vi "SDG60CreateArbWaveformFlatten3.vi"(4 "WFM Source":u16(ring) items=["Single file", "Split files", "Array"], 5 "WFM (Column) Number":i32, 6 "Array WFM":i16[](array[numeric])=[1000, 2000, 3000, 4000, 5000, 6000, 7000, 8000], 7 "WFM Length":i32=15, 8 "error in (no error)":errorcluster, 9 "Timeout (40000 ms)":u32=40000, 10 "Waveform Name (\"wave1\")":string="wave1", 11 "VISA resource name":refnum<visa-resource-name>="USB0::0xF4EC::0x1101::SDG6XEBC5R0119::INSTR") -> (0 "error out":errorcluster, 3 "VISA resource name out":refnum<visa-resource-name>)   [LabVIEW 2018]
doc: "Creates and saves an arbitrary (user-defined) waveform in non-volatile memory, then selects it for output."
uses:
  <vilib>/Utility/file.llb/Read From Spreadsheet File (I64).vi
panel:
  out "Check String":string
  out "WFM to arr time":dbl
  out "Arr to str time":dbl
  out "Upload time":dbl
  out "Total time":dbl
  out "Attempts 0: First":i32
  in  "WFM Path":path=path "C:/Data/_SoftDevelopment/SDG6000/WFMTst20E6PtsInt.txt"
  # "Same vi as with suppliers example, but incorrect negative case removed.\nInstead calculating twos complement explicitly for negative values.\nThe input range for ARB data is: -32767..+32767 (must be integers)\n\nC1 hardcoded as needs to have a channel\nassigned to be uploaded. \nCan then be selected for either channel\n\nUpon overwrite of name with new WFM, still needs to be selected\notherwise will still use old WFM. If WFM has been selected, and then gets deleted off \nC drive, will still output WFM on that channel\n\nTesting uploads of large WFMS.\n8M: All ok, can have 2 separate WFMs on 2 channels and upload more\n16M: Can have 2 separate WFMs on 2 channels, storage space limits 3rd upload\n          of 16M points, but can upload 8M and switch fine between them all.\n20M: Can have 20M on both channels, but then no storage space to upload third\n\nVi will write the file with a small (16B bin file on device) file (overwriting any WFM \n           preciviously with that name),  then write the WFM selected with the one chosen to \n           upload.  This means you don't need to clear space off the device, as long as the \n           name of the WFM is already on the device. Provided it is that file that is the storage \n           issue. If a new name is chosen, then will have to manually delete the old WFM.\n\nIf too large a waveform is uploaded, generator will crash requiring manual power cycle\n\nIf storage full, will beep on machine-say storage full, but not give any error through \nlabview. Waveform won't ovewrite others when uploading\n\nSingle pixel test, (osciiloscope limited), for 20M points, the single pixel did go high, Pk-Pk on \nscope was 3.6V when should be 4.0 Vpp. This may be down to the scopes 200MHz resolution\nas the width of the of peak on the scope is ~350ns"
  # "Need to set name to be number. not string"
  # "Max  20E6 (decimal)"
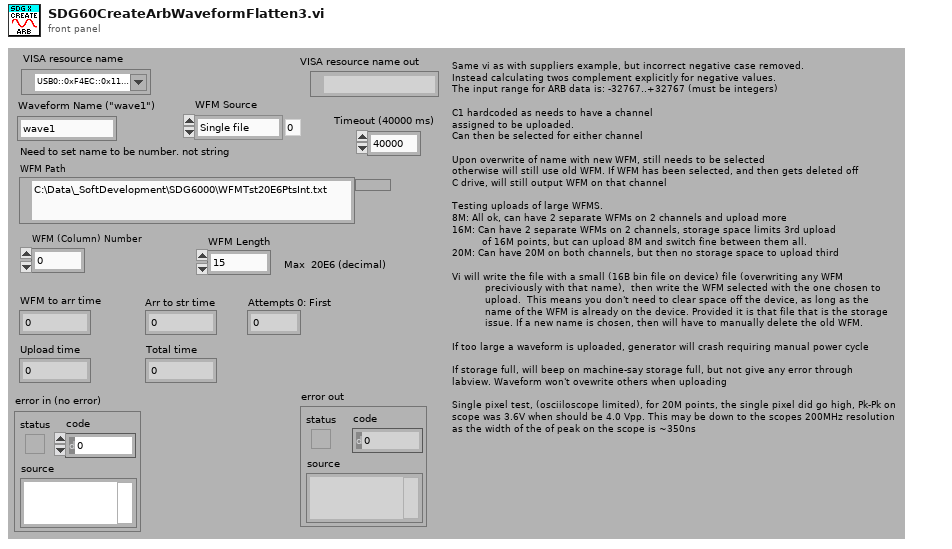
[diagram p1: front panel]
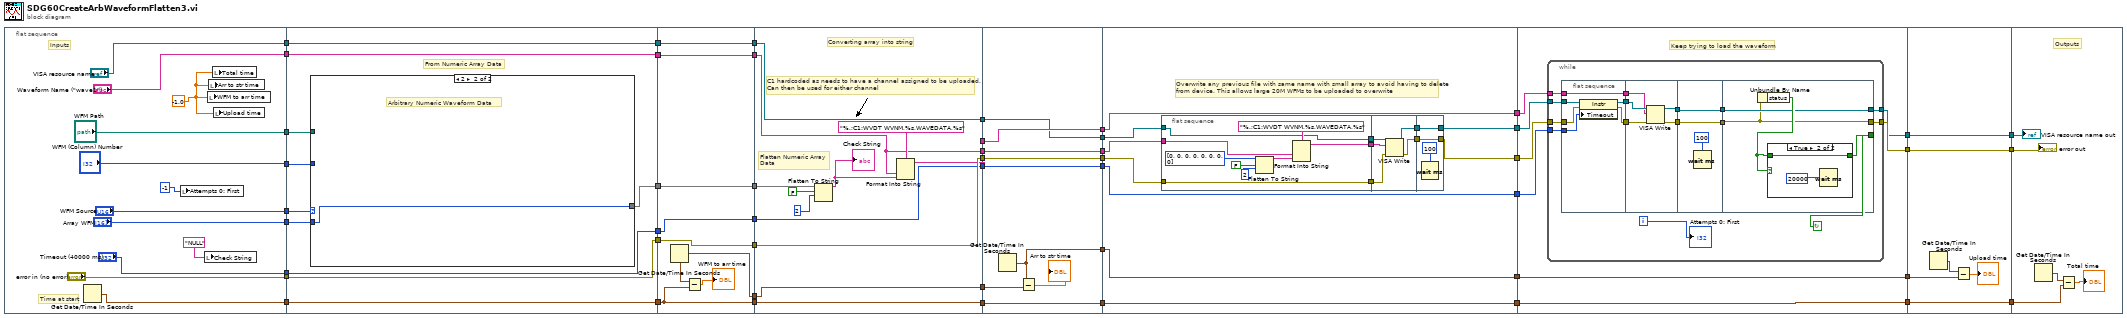
[diagram p0: block diagram]
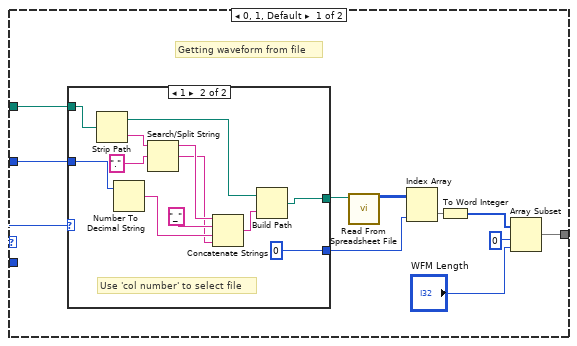
[diagram p2: hidden frame]
diagram:
  n1 = flat-sequence {
    tunnel: ["WFM Source"] -> w49
    tunnel: ["Array WFM"] -> w48
    tunnel: ["WFM Path"] -> w47
    tunnel: ["WFM (Column) Number"] -> w46
    tunnel: ["VISA resource name"] -> w45
    tunnel: ["Waveform Name (\"wave1\")"] -> w44
    tunnel: ["error in (no error)"] -> w43
    tunnel: ["Timeout (40000 ms)"] -> w42
    tunnel: [w53] -> w41
    tunnel: w49 -> [w71]
    tunnel: w48 -> [w70]
    tunnel: [w69] -> w40
    tunnel: w47 -> [w68]
    tunnel: w46 -> [w67]
    tunnel: [w66] -> w38
    tunnel: w45 -> [w66]
    tunnel: [w65] -> w36
    tunnel: w44 -> [w65]
    tunnel: [w64] -> w34
    tunnel: w43 -> [w64]
    tunnel: [w63] -> w32
    tunnel: w42 -> [w63]
    tunnel: [w62] -> w30
    tunnel: w41 -> [w62]
    tunnel: w40 -> [w105]
    tunnel: [w105] -> w39
    tunnel: w38 -> [w104]
    tunnel: [w104] -> w37
    tunnel: w36 -> [w103]
    tunnel: [w103] -> w35
    tunnel: w34 -> [w99]
    tunnel: [w99] -> w33
    tunnel: w32 -> [w100]
    tunnel: [w100] -> w31
    tunnel: w30 -> [w101]
    tunnel: [w101] -> w29
    tunnel: [w98] -> w15
    tunnel: w39 -> [w109]
    tunnel: [w111] -> w28
    tunnel: [w116] -> w27
    tunnel: [w115] -> w26
    tunnel: [w114] -> w25
    tunnel: w37 -> [w116]
    tunnel: w35 -> [w106]
    tunnel: w33 -> [w115]
    tunnel: w31 -> [w114]
    tunnel: w29 -> [w113]
    tunnel: [w113] -> w24
    tunnel: [w112] -> w16
    tunnel: w15 -> [w112]
    tunnel: [w106] -> w1
    tunnel: w28 -> [w126]
    tunnel: [w126] -> w14
    tunnel: w27 -> [w125]
    tunnel: [w125] -> w12
    tunnel: w26 -> [w124]
    tunnel: [w124] -> w10
    tunnel: w25 -> [w123]
    tunnel: [w123] -> w8
    tunnel: w24 -> [w119]
    tunnel: [w119] -> w6
    tunnel: [w121] -> w4
    tunnel: w16 -> [w120]
    tunnel: [w118] -> w2
    tunnel: w1 -> [w118]
    tunnel: w14 -> [w140]
    tunnel: [w140] -> w13
    tunnel: w12 -> [w128]
    tunnel: [w127] -> w11
    tunnel: w10 -> [w132]
    tunnel: [w131] -> w9
    tunnel: w8 -> [w139]
    tunnel: [w139] -> w7
    tunnel: w6 -> [w138]
    tunnel: [w138] -> w5
    tunnel: w4 -> [w137]
    tunnel: [w137] -> w3
    tunnel: w2 -> [w136]
    tunnel: [w161] -> w23
    tunnel: [w160] -> w21
    tunnel: w13 -> [w165]
    tunnel: w11 -> [w164]
    tunnel: w9 -> [w163]
    tunnel: w7 -> [w162]
    tunnel: w5 -> [w159]
    tunnel: [w159] -> w19
    tunnel: w3 -> [w158]
    tunnel: [w158] -> w17
    tunnel: w23 -> [w207]
    tunnel: [w207] -> w22
    tunnel: w21 -> [w206]
    tunnel: [w206] -> w20
    tunnel: w19 -> [w204]
    tunnel: [w204] -> w18
    tunnel: w17 -> [w203]
    tunnel: w22 -> [w212]
    tunnel: w20 -> [w211]
    tunnel: w18 -> [w208]
    frame #0 {
      w52 = -1.0
      # "Inputs"
      # "Time at start"
      n2 = Get Date/Time In Seconds() -> (seconds since 1Jan1904=w53:timestamp)
      n3 = local write "Attempts 0: First"(-1) -> ()
      n4 = local write "Check String"("NULL") -> ()
      n5 = local write "WFM to arr time"(w52) -> ()
      n6 = local write "Arr to str time"(w52) -> ()
      n7 = local write "Total time"(w52) -> ()
      n8 = local write "Upload time"(w52) -> ()
    }
    frame #1 {
      # "From Numeric Array Data"
      n9 = case shown="2" w71 {
        selector: w71 -> [w80 _]
        tunnel: [w75 w97] -> w69
        tunnel: w70 -> [_ w97]
        tunnel: w68 -> [w74 _]
        tunnel: w67 -> [w73 _]
        frame 0, 1, Default {
          # "Getting waveform from file"
          n10 = case shown="1" w80 {
            tunnel: w74 -> [w84 w96]
            tunnel: w73 -> [w83 w93]
            tunnel: [w84 w86] -> w78
            tunnel: [w83 0 ("x")] -> w77
            frame 0, Default {
              # "File contains multiple wfms"
            }
            frame 1 {
              # "Use 'col number' to select file"
              n11 = Strip Path(path=w96) -> (stripped path=w88:path, name=w94:string)
              n12 = Number To Decimal String(number=w93) -> (decimal integer string=w90:string)  [unwired: 1 in]
              n13 = Search/Split String(string=w94, search string/char (-)=".") -> (substring before match=w92:string, match + rest of string=w89:string)  [unwired: 1 in, 1 out]
              n14 = Concatenate Strings(w92, "_", w90, w89) -> (w87:string)
              n15 = Build Path(base path=w88, name or relative path=w87) -> (appended path=w86:path)
            }
          }
          n16 = call-poly <vilib>:"Read From Spreadsheet File.vi"("file path (dialog if empty)"=w78) -> ("all rows"=w79:i64[][])  [unwired: 6 in, 4 out]
          n17 = Index Array(array=w79, index (col)=w77) -> (element=w76:i64[])  [unwired: 1 in]
          n18 = To Word Integer(number=w76) -> (16bit integer=w82:i16[])
          n19 = Array Subset(array=w82, index=0 ("x"), length="WFM Length") -> (w75:i16[])
        }
        frame 2 {
          # "Arbitrary Numeric Waveform Data"
        }
      }
    }
    frame #2 {
      n20 = Get Date/Time In Seconds() -> (seconds since 1Jan1904=w98:timestamp)
      n21 = Subtract(x=w98, y=w101) -> (x-y=→"WFM to arr time":dbl)
    }
    frame #3 {
      # "Converting array into string"
      # "C1 hardcoded as needs to have a channel assigned to be uploaded. \nCan then be used for either channel"
      # "Flatten Numeric Array \nData"
      n22 = Flatten To String(anything=w109, prepend array or string size? (T)=FALSE, byte order (0:big-endian, network order)=2) -> (data string=w107:string)  [unwired: 1 in, 2 out]
      "Check String" <- w107
      n23 = Format Into String(format string="%.;C1:WVDT WVNM,%s,WAVEDATA,%s", w106, w107) -> (resulting string=w111:string)  [unwired: 2 in, 1 out]
    }
    frame #4 {
      n24 = Get Date/Time In Seconds() -> (seconds since 1Jan1904=w121:timestamp)
      n25 = Subtract(x=w121, y=w120) -> (x-y=→"Arr to str time":dbl)
    }
    frame #5 {
      # "Overwrite any previous file with same name with small array to avoid having to delete\nfrom device. This allows large 20M WFMs to be uploaded to overwrite"
      n26 = flat-sequence {
        tunnel: w136 -> [w148]
        tunnel: [w143] -> w135
        tunnel: w132 -> [w142]
        tunnel: [w142] -> w134
        tunnel: w128 -> [w141]
        tunnel: [w141] -> w130
        tunnel: w135 -> [w154]
        tunnel: w134 -> [w153]
        tunnel: [w152] -> w133
        tunnel: w130 -> [w151]
        tunnel: [w150] -> w129
        tunnel: [w156] -> w131
        tunnel: w133 -> [w156]
        tunnel: [w155] -> w127
        tunnel: w129 -> [w155]
        frame #0 {
          n27 = Flatten To String(anything=i16[] [0, 0, 0, 0, 0, 0, 0, 0] ("Array WFM DUMMY"), prepend array or string size? (T)=FALSE, byte order (0:big-endian, network order)=2) -> (data string=w145:string)  [unwired: 1 in, 2 out]
          n28 = Format Into String(format string="%.;C1:WVDT WVNM,%s,WAVEDATA,%s", w148, w145) -> (resulting string=w143:string)  [unwired: 2 in, 1 out]
        }
        frame #1 {
          n29 = VISA Write(VISA resource name=w151, write buffer=w154, error in (no error)=w153) -> (VISA resource name out=w150:refnum<visa-resource-name>, error out=w152:errorcluster)  [unwired: 1 out]
        }
        frame #2 {
          n30 = Wait (ms)(milliseconds to wait=100 ("x")) -> ()  [unwired: 1 out]
        }
      }
    }
    frame #6 {
      # "Keep trying to load the waveform"
      n31 = while {
        tunnel: w165 -> [w180]
        tunnel: w164 -> [w179]
        tunnel: w163 -> [w178]
        tunnel: [w177] -> w161
        tunnel: [w176] -> w160
        tunnel: w162 -> [w166]
        i -> [w172]
        stop <- w175 continue-if-true
        n32 = flat-sequence {
          tunnel: w180 -> [w186]
          tunnel: w178 -> [w183]
          tunnel: w179 -> [w185]
          tunnel: [w184] -> w169
          tunnel: [w182] -> w168
          tunnel: [w186] -> w167
          tunnel: w166 -> [w181]
          tunnel: [w187] -> w174
          tunnel: [w188] -> w173
          tunnel: w169 -> [w190]
          tunnel: w168 -> [w191]
          tunnel: w167 -> [w189]
          tunnel: w174 -> [w192]
          tunnel: w173 -> [w193]
          tunnel: [w193] -> w171
          tunnel: [w192] -> w170
          tunnel: [w196] -> w176
          tunnel: [w195] -> w177
          tunnel: [w197] -> w175
          tunnel: w171 -> [w196]
          tunnel: w170 -> [w195]
          frame #0 {
            n33 = property class="Instr"(reference=w185, error in=w183, "Timeout"=w181) -> (reference out=w184:refnum<visa-resource-name>, error out=w182:errorcluster)
          }
          frame #1 {
            n34 = VISA Write(VISA resource name=w190, write buffer=w189, error in (no error)=w191) -> (VISA resource name out=w188:refnum<visa-resource-name>, error out=w187:errorcluster)  [unwired: 1 out]
          }
          frame #2 {
            n35 = Wait (ms)(milliseconds to wait=100 ("x")) -> ()  [unwired: 1 out]
          }
          frame #3 {
            n36 = Unbundle By Name(w195) -> ("status"=w198:bool)
            n37 = case shown="True" w198 {
              tunnel: w198 -> [w199 w200]
              tunnel: [w199 w200] -> w197
              frame False {
              }
              frame True {
                n38 = Wait (ms)(milliseconds to wait=20000 ("x")) -> ()  [unwired: 1 out]
              }
            }
          }
        }
        "Attempts 0: First" <- w172
      }
    }
    frame #7 {
      n39 = Get Date/Time In Seconds() -> (seconds since 1Jan1904=w205:timestamp)
      n40 = Subtract(x=w205, y=w203) -> (x-y=→"Upload time":dbl)
    }
    frame #8 {
      # "Outputs"
      n41 = Get Date/Time In Seconds() -> (seconds since 1Jan1904=w210:timestamp)
      n42 = Subtract(x=w210, y=w208) -> (x-y=→"Total time":dbl)
      "VISA resource name out" <- w211
      "error out" <- w212
    }
  }
